vi "Write Average.vi"(8 "error in (no error)":errorcluster, 10 "Average":dbl, 11 "Averager in":refnum<class "Averager.lvclass">) -> (0 "error out":errorcluster, 3 "Averager out":refnum<class "Averager.lvclass">)   [LabVIEW 2018, in "Averager.lvclass"]
uses:
  Averager.lvclass
  Averager.lvclass/Averager.ctl
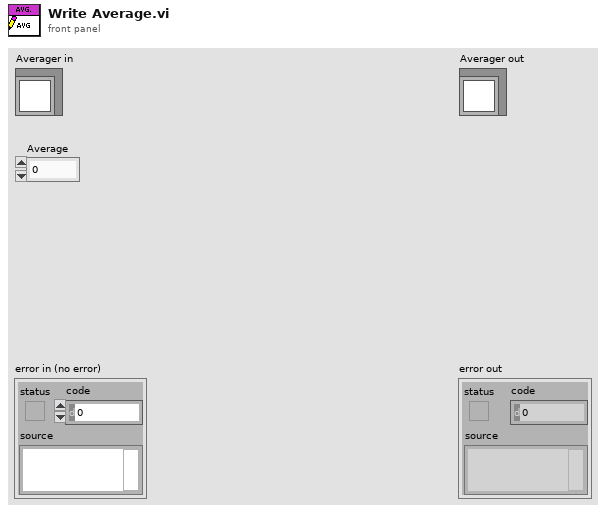
[diagram p1: front panel]
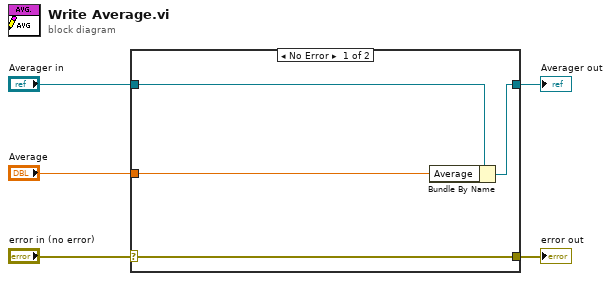
[diagram p0: block diagram]
diagram:
  n1 = case shown="No Error" "error in (no error)" {
    selector: "error in (no error)" -> [w9 w10]
    tunnel: [w9 w10] -> w4
    tunnel: [w7 w11] -> w2
    tunnel: "Averager in" -> [w8 w11]
    tunnel: "Average" -> [w6 _]
    frame No Error {
      n2 = Bundle By Name(cluster=w8, "Average"=w6) -> (w7:refnum<class "Averager.lvclass">)
    }
    frame Error {
    }
  }
  "error out" <- w4
  "Averager out" <- w2
